vi "test Parse Simple Array.vi"() -> (0 "error out":errorcluster, 2 "pass?":bool)   [LabVIEW 2019, in "RESP3 Tests.lvlib"]
uses:
  RESP3 Tests.lvlib
  RESP3/RESP3 Parser/RESP3 Parser.lvclass
  RESP3/types/RESP3 Type.ctl
  RESP3/types/RESP3 data type attribute.vi
  RESP3/RESP3.lvlib
panel:
  out "RESP3 Value":variant
  out "finished?":bool
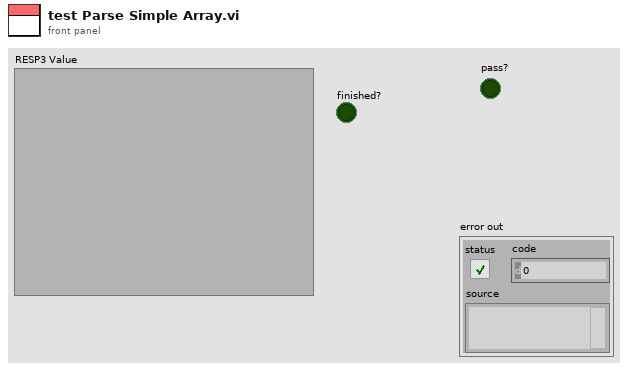
[diagram p1: front panel]
types:
  T1 = typedef "RESP3.lvlib/RESP3 Type.ctl" = enum8{"<0x00>", "<0x01>", "<0x02>", "<0x03>", "<0x04>", "<0x05>", "<0x06>", "<0x07>", "<0x08>", "<0x09>", "<0x0A>", "<0x0B>", "<0x0C>", "<0x0D>", "<0x0E>", "<0x0F>", "<0x10>", "<0x11>", "<0x12>", "<0x13>", "<0x14>", "<0x15>", "<0x16>", "<0x17>", "<0x18>", "<0x19>", "<0x1A>", "<0x1B>", "<0x1C>", "<0x1D>", "<0x1E>", "<0x1F>", "\" \"", "BLOB ERROR", "\"\"\"", "BOOLEAN", "BLOB", "MAP", "\"&\"", "\"'\"", "BIG NUMBER", "\")\"", "ARRAY", "STRING", "DOUBLE", "ERROR", "END", "\"/\"", "\"0\"", "\"1\"", "\"2\"", "\"3\"", "\"4\"", "\"5\"", "\"6\"", "\"7\"", "\"8\"", "\"9\"", "INTEGER", "STREAM", "\"<\"", "VERBATIM STRING", "PUSH", "\"?\"", "\"@\"", "\"A\"", "\"B\"", "\"C\"", "\"D\"", "\"E\"", "\"F\"", "\"G\"", "\"H\"", "\"I\"", "\"J\"", "\"K\"", "\"L\"", "\"M\"", "\"N\"", "\"O\"", "\"P\"", "\"Q\"", "\"R\"", "\"S\"", "\"T\"", "\"U\"", "\"V\"", "\"W\"", "\"X\"", "\"Y\"", "\"Z\"", "\"[\"", "\"\\\"", "\"]\"", "\"^\"", "NULL", "\"`\"", "\"a\"", "\"b\"", "\"c\"", "\"d\"", "\"e\"", "\"f\"", "\"g\"", "\"h\"", "\"i\"", "\"j\"", "\"k\"", "\"l\"", "\"m\"", "\"n\"", "\"o\"", "\"p\"", "\"q\"", "\"r\"", "\"s\"", "\"t\"", "\"u\"", "\"v\"", "\"w\"", "\"x\"", "\"y\"", "\"z\"", "\"{\"", "ATTRIBUTES", "\"}\"", "SET", "<0x7F>", "<0x80>", "<0x81>", "<0x82>", "<0x83>", "<0x84>", "<0x85>", "<0x86>", "<0x87>", "<0x88>", "<0x89>", "<0x8A>", "<0x8B>", "<0x8C>", "<0x8D>", "<0x8E>", "<0x8F>", "<0x90>", "<0x91>", "<0x92>", "<0x93>", "<0x94>", "<0x95>", "<0x96>", "<0x97>", "<0x98>", "<0x99>", "<0x9A>", "<0x9B>", "<0x9C>", "<0x9D>", "<0x9E>", "<0x9F>", "<0xA0>", "<0xA1>", "<0xA2>", "<0xA3>", "<0xA4>", "<0xA5>", "<0xA6>", "<0xA7>", "<0xA8>", "<0xA9>", "<0xAA>", "<0xAB>", "<0xAC>", "<0xAD>", "<0xAE>", "<0xAF>", "<0xB0>", "<0xB1>", "<0xB2>", "<0xB3>", "<0xB4>", "<0xB5>", "<0xB6>", "<0xB7>", "<0xB8>", "<0xB9>", "<0xBA>", "<0xBB>", "<0xBC>", "<0xBD>", "<0xBE>", "<0xBF>", "<0xC0>", "<0xC1>", "<0xC2>", "<0xC3>", "<0xC4>", "<0xC5>", "<0xC6>", "<0xC7>", "<0xC8>", "<0xC9>", "<0xCA>", "<0xCB>", "<0xCC>", "<0xCD>", "<0xCE>", "<0xCF>", "<0xD0>", "<0xD1>", "<0xD2>", "<0xD3>", "<0xD4>", "<0xD5>", "<0xD6>", "<0xD7>", "<0xD8>", "<0xD9>", "<0xDA>", "<0xDB>", "<0xDC>", "<0xDD>", "<0xDE>", "<0xDF>", "<0xE0>", "<0xE1>", "<0xE2>", "<0xE3>", "<0xE4>", "<0xE5>", "<0xE6>", "<0xE7>", "<0xE8>", "<0xE9>", "<0xEA>", "<0xEB>", "<0xEC>", "<0xED>", "<0xEE>", "<0xEF>", "<0xF0>", "<0xF1>", "<0xF2>", "<0xF3>", "<0xF4>", "<0xF5>", "<0xF6>", "<0xF7>", "<0xF8>", "<0xF9>", "<0xFA>", "<0xFB>", "<0xFC>", "<0xFD>", "<0xFE>"}
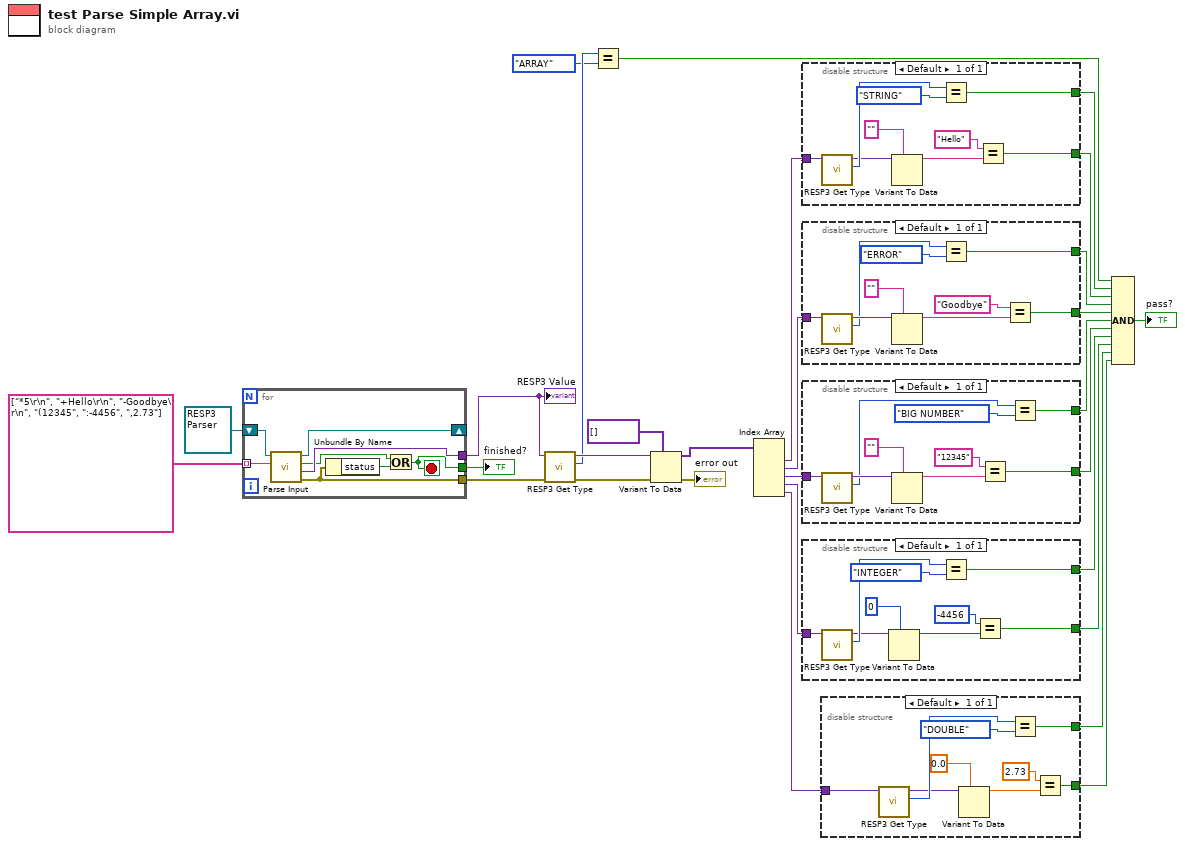
[diagram p0: block diagram]
diagram:
  n1 = for {
    shift-right: [w35] -> _
    shift-left: refnum<class "RESP3 Parser.lvclass"> refnum ("RESP3.lvlib:RESP3 Parser.lvclass") -> [w36]
    tunnel: string[] ["*5\r\n", "+Hello\r\n", "-Goodbye\r\n", "(12345", ":-4456", ",2.73"] -> [w34] mode=indexing
    tunnel: [w33] -> w24
    tunnel: [w31] -> w26
    tunnel: [w29] -> w19
    stop <- w31 stop-if-true
    n2 = call-dynamic "Parse Input.vi"("input line"=w34, "RESP3 Parser in"=w36) -> ("error out"=w29:errorcluster, "RESP3 Value"=w33:variant, "finished?"=w32:bool, "RESP3 Parser out"=w35:refnum<class "RESP3 Parser.lvclass">)  [unwired: 6 in]
    n3 = Unbundle By Name(w29) -> ("status"=w30:bool)
    n4 = Or(x=w32, y=w30) -> (x .or. y?=w31:bool)
  }
  "finished?" <- w26
  "RESP3 Value" <- w24
  n5 = call "RESP3 Get Type.vi"("RESP3 Value in"=w24) -> ("RESP3 Type"=w22:T1, "RESP3 Value out"=w23:variant)  [unwired: 7 in, 2 out]
  n6 = Equal?(x=w22, y=RESP3_Type."ARRAY") -> (x = y?=w20:bool)
  n7 = Variant To Data(error in=w19, type=variant[] [], Variant=w23) -> (data=w18:variant[], error out=→"error out":errorcluster)
  n8 = Index Array(array=w18) -> (element #1=w17:variant, element #2=w14:variant, element #3=w10:variant, element #4=w5:variant, element #5=w6:variant)  [unwired: 5 in]
  n9 = disable-structure shown="Default" {
    disable-tunnel: w17 -> [w45]
    disable-tunnel: [w42] -> w16
    disable-tunnel: [w37] -> w15
    frame Enabled {
      n10 = call "RESP3 Get Type.vi"("RESP3 Value in"=w45) -> ("RESP3 Type"=w43:T1, "RESP3 Value out"=w41:variant)  [unwired: 7 in, 2 out]
      n11 = Variant To Data(type="", Variant=w41) -> (data=w39:string)  [unwired: 1 in, 1 out]
      n12 = Equal?(x=w43, y=RESP3_Type."STRING") -> (x = y?=w42:bool)
      n13 = Equal?(x="Hello", y=w39) -> (x = y?=w37:bool)
    }
  }
  n14 = disable-structure shown="Default" {
    disable-tunnel: w14 -> [w48]
    disable-tunnel: [w47] -> w13
    disable-tunnel: [w46] -> w12
    frame Enabled {
      n15 = call "RESP3 Get Type.vi"("RESP3 Value in"=w48) -> ("RESP3 Type"=w51:T1, "RESP3 Value out"=w52:variant)  [unwired: 7 in, 2 out]
      n16 = Variant To Data(type="", Variant=w52) -> (data=w53:string)  [unwired: 1 in, 1 out]
      n17 = Equal?(x=w51, y=RESP3_Type."ERROR") -> (x = y?=w47:bool)
      n18 = Equal?(x="Goodbye", y=w53) -> (x = y?=w46:bool)
    }
  }
  n19 = disable-structure shown="Default" {
    disable-tunnel: w10 -> [w57]
    disable-tunnel: [w56] -> w9
    disable-tunnel: [w55] -> w8
    frame Enabled {
      n20 = call "RESP3 Get Type.vi"("RESP3 Value in"=w57) -> ("RESP3 Type"=w60:T1, "RESP3 Value out"=w61:variant)  [unwired: 7 in, 2 out]
      n21 = Variant To Data(type="", Variant=w61) -> (data=w62:string)  [unwired: 1 in, 1 out]
      n22 = Equal?(x="12345", y=w62) -> (x = y?=w55:bool)
      n23 = Equal?(x=w60, y=RESP3_Type."BIG NUMBER") -> (x = y?=w56:bool)
    }
  }
  n24 = disable-structure shown="Default" {
    disable-tunnel: [w70] -> w4
    disable-tunnel: [w64] -> w3
    disable-tunnel: w5 -> [w68]
    frame Enabled {
      n25 = call "RESP3 Get Type.vi"("RESP3 Value in"=w68) -> ("RESP3 Type"=w71:T1, "RESP3 Value out"=w69:variant)  [unwired: 7 in, 2 out]
      n26 = Variant To Data(type=i64 0, Variant=w69) -> (data=w66:i64)  [unwired: 1 in, 1 out]
      n27 = Equal?(x=w71, y=RESP3_Type."INTEGER") -> (x = y?=w70:bool)
      n28 = Equal?(x=i64 -4456, y=w66) -> (x = y?=w64:bool)
    }
  }
  n29 = disable-structure shown="Default" {
    disable-tunnel: [w79] -> w2
    disable-tunnel: [w73] -> w1
    disable-tunnel: w6 -> [w77]
    frame Enabled {
      n30 = call "RESP3 Get Type.vi"("RESP3 Value in"=w77) -> ("RESP3 Type"=w80:T1, "RESP3 Value out"=w78:variant)  [unwired: 7 in, 2 out]
      n31 = Variant To Data(type=0.0, Variant=w78) -> (data=w75:dbl)  [unwired: 1 in, 1 out]
      n32 = Equal?(x=w80, y=RESP3_Type."DOUBLE") -> (x = y?=w79:bool)
      n33 = Equal?(x=2.73, y=w75) -> (x = y?=w73:bool)
    }
  }
  n34 = Compound Arithmetic op=AND(w20, w16, w15, w13, w12, w9, w8, w4, w3, w2, w1) -> (→"pass?":bool)
